vi "Redirection Collection.vi"(8 "error in":errorcluster) -> (0 "error out":errorcluster)   [LabVIEW 2020, in "MainVIs.lvlib"]
uses:
  MainVIs.lvlib
  <vilib>/Utility/miscctls.llb/LVCursorListTypeDef.ctl
  Collection Support/Controls/PED States.ctl
  Collection Support/Controls/FirstCall.ctl
  CollectionSupport.lvlib
panel:
  in  "Delay":u32 max=1000 step=50
  in  "Trial Duration (s)":dbl=10.0 format="%#_13g"
  in  "Max Time":dbl=1.3 min=0.0 max=2.0 format="%#_13g"
  in  "Min Time":dbl=0.8 min=0.0 max=1.0 step=0.1 format="%#_13g"
  in  "Start Second":dbl=2.5 min=1.0 max=2.5 step=0.1 format="%#_13g"
  in  "Interruptions":i32
  in  "Settings":bool
  in  "Restart Button":bool
  in  "Exit Button":bool
  out "Flow Chart":dynamicdata(graph)
  out "Audio Chart":dynamicdata(graph)
  in  "START/STOP":bool
  out "GO/STOP":bool
  out "SPL Chart":cluster{"Y":dbl[], "Y":dbl[]}[](graph)
  out "Countdown":dbl format="%#.0g"
  out "Pressure Chart":dynamicdata(graph)
  in  "Stopped?":bool
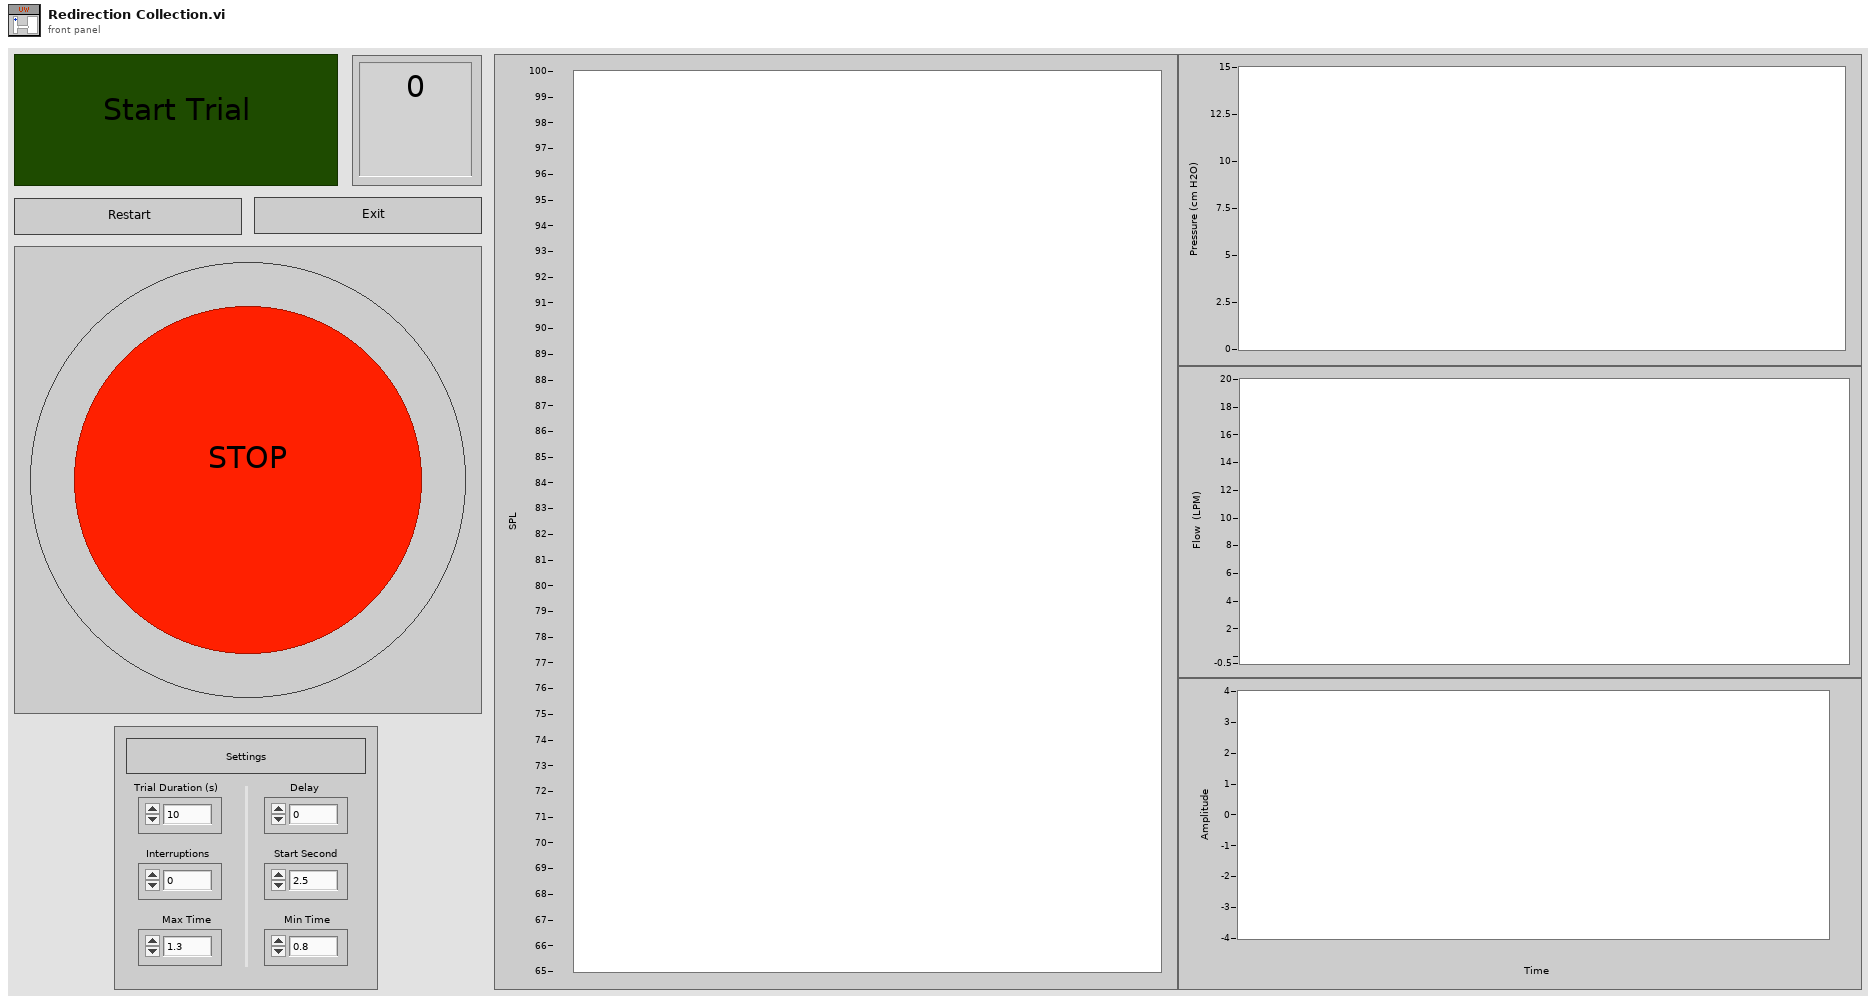
[diagram p1: front panel]
types:
  T1 = enum16{"open", "replace", "create", "open or create", "replace or create", "replace or create with confirmation"}
  T2 = typedef "LVCursorListTypeDef.ctl" = cluster{"Name":string, "Color":u32, "Style":u8, "Point Style":u8, "Name Visible":bool, "Allow Drag":bool, "Cursor Mode":u32, "Plot":i32, "Index":i32, "Position":cluster{"X":dbl, "Y":dbl}, "X Scale":u32, "Y Scale":u32, "Watch Plots":i32[], "Watch All Plots":bool, "Plot Area":i32, "Label Offset":cluster{"X":dbl, "Y":dbl}}[]
  T3 = typedef "CollectionSupport.lvlib/PED States.ctl" = enum16{"Initialize", "Wait", "Record", "Save", "Reset", "Exit"}
  T4 = typedef "CollectionSupport.lvlib/FirstCall.ctl" = enum16{"First", "After"}
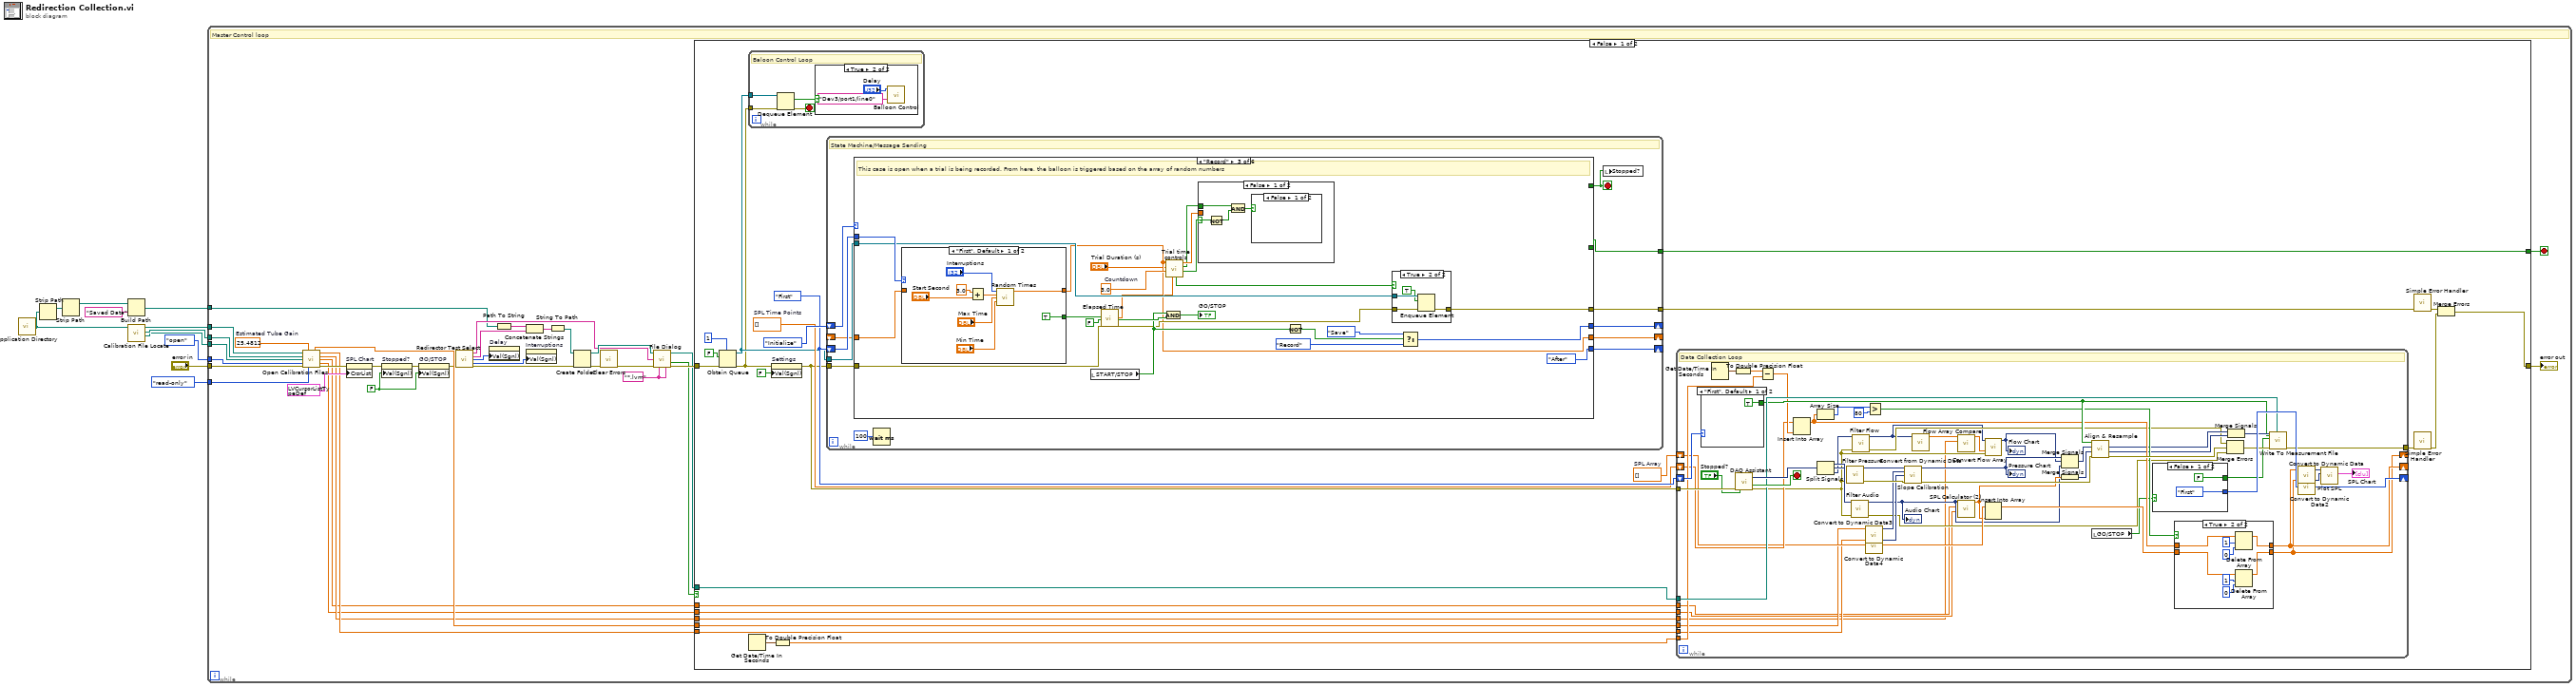
[diagram p0: block diagram]
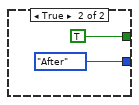
[diagram p4: hidden frame]
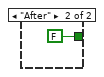
[diagram p5: hidden frame]
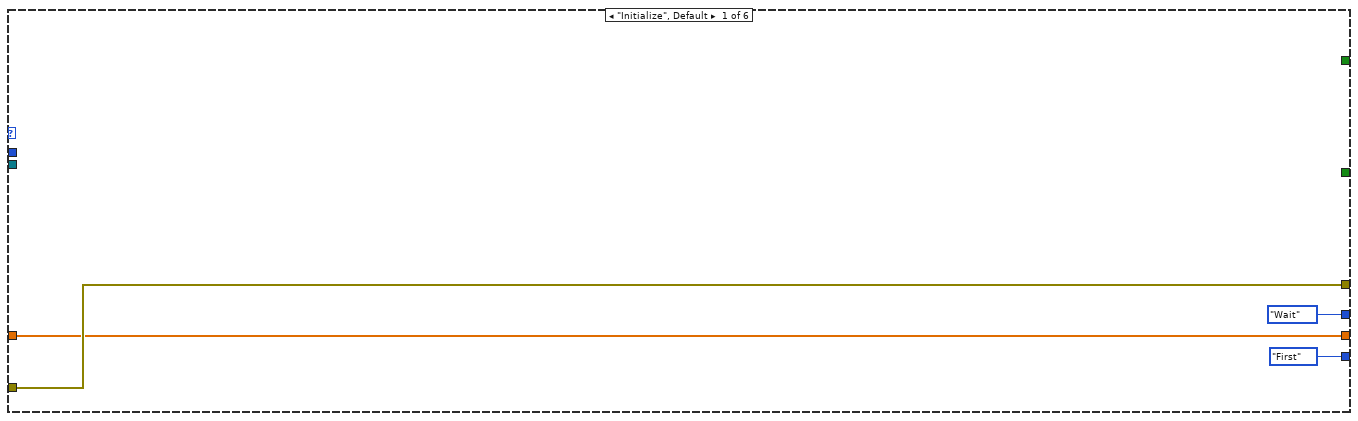
[diagram p6: hidden frame]
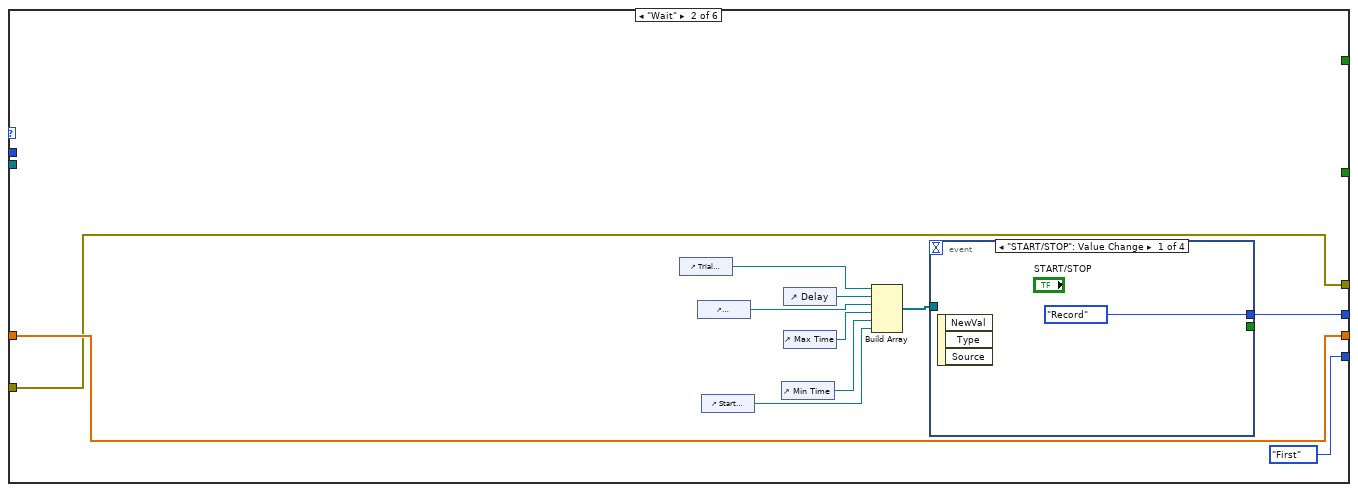
[diagram p7: hidden frame]
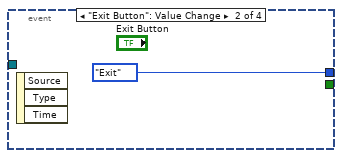
[diagram p8: hidden frame]
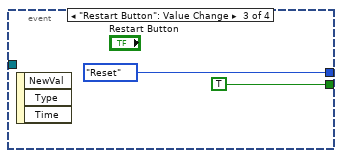
[diagram p9: hidden frame]
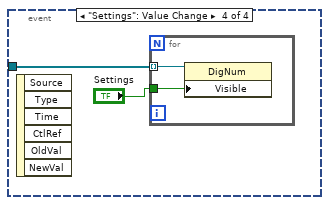
[diagram p10: hidden frame]
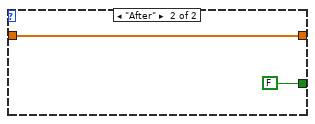
[diagram p12: hidden frame]
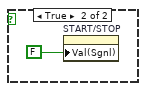
[diagram p13: hidden frame]
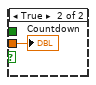
[diagram p14: hidden frame]
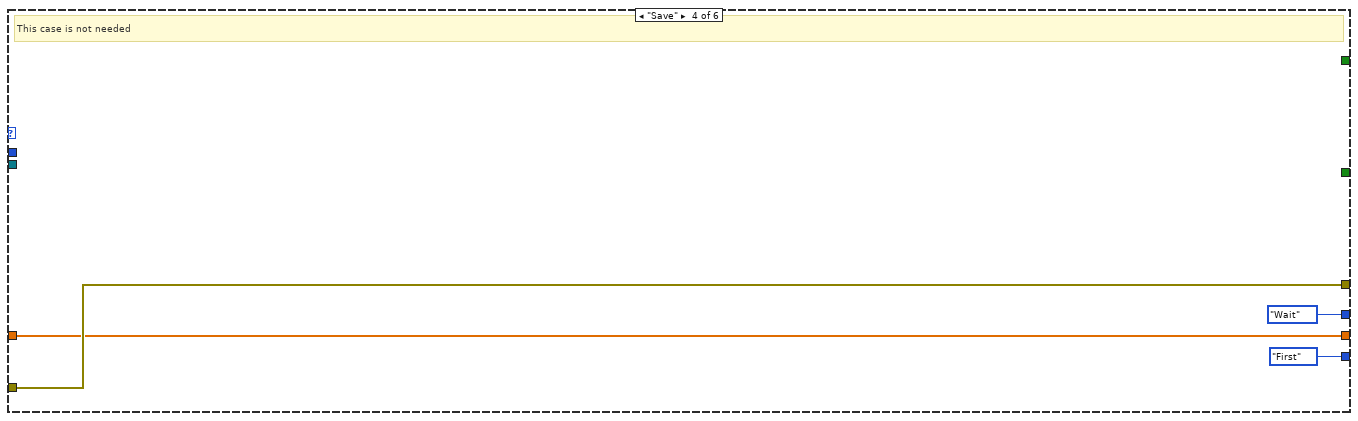
[diagram p15: hidden frame]
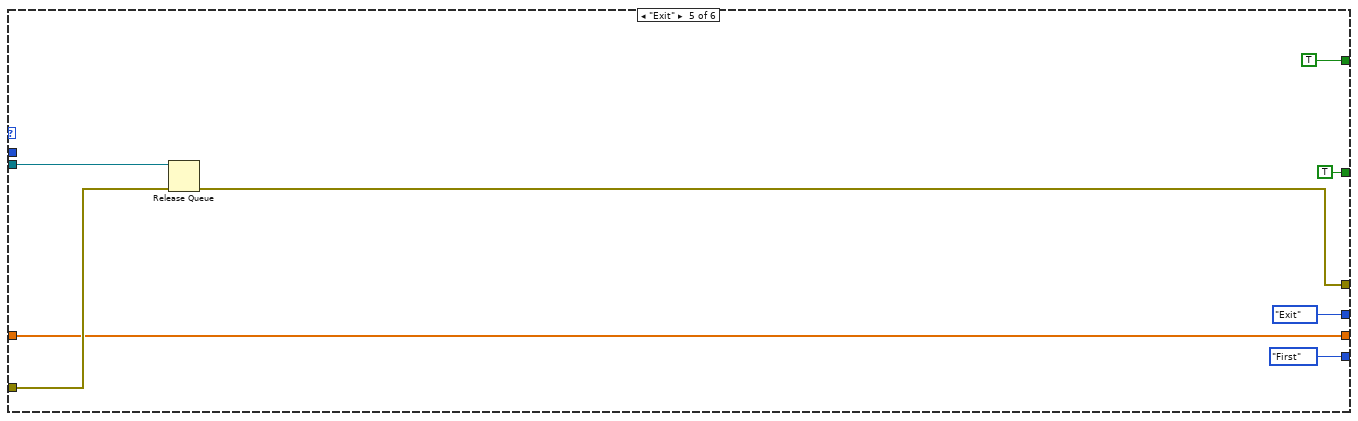
[diagram p16: hidden frame]
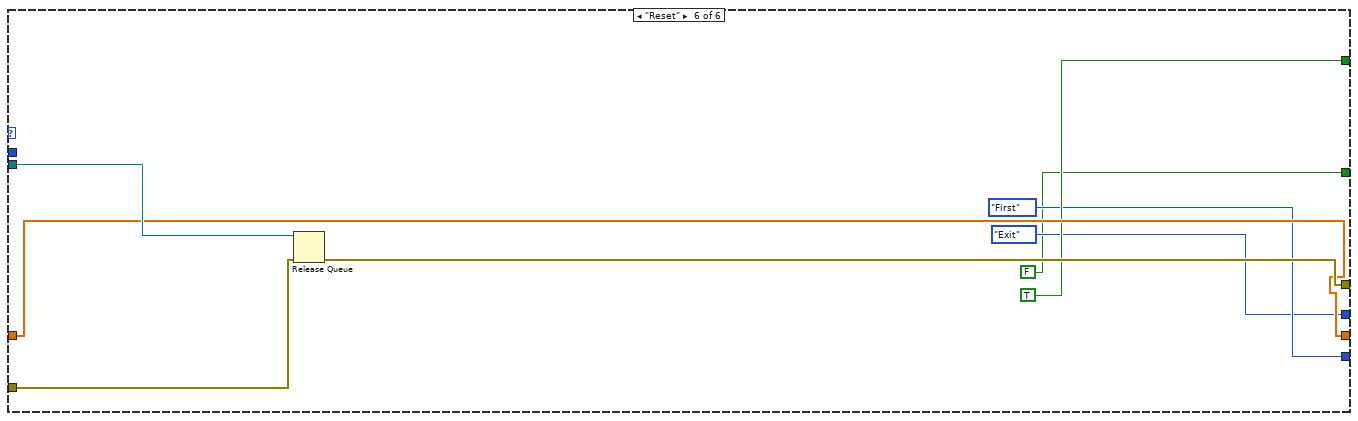
[diagram p17: hidden frame]
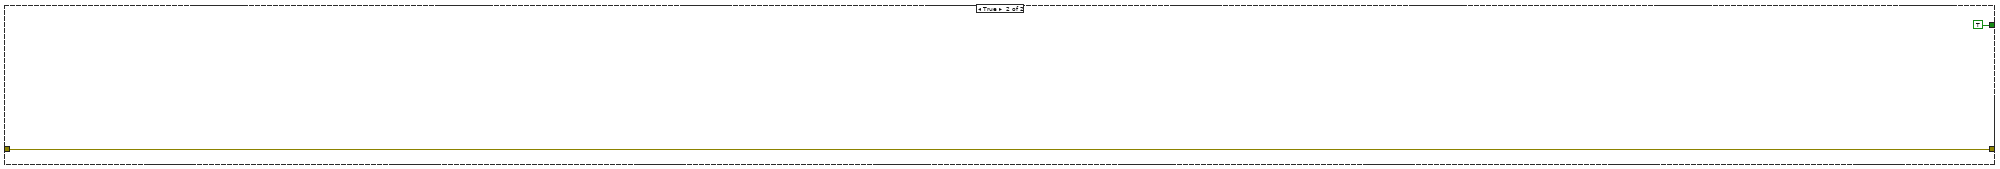
[diagram p18: hidden frame]
diagram:
  n1 = call <vilib>:"Application Directory.vi"() -> ("Application Directory"=w3:path)
  n2 = Strip Path(path=w3) -> (stripped path=w8:path)  [unwired: 1 out]
  n3 = Strip Path(path=w8) -> (stripped path=w2:path)  [unwired: 1 out]
  n4 = Build Path(base path=w2, name or relative path="Saved Data") -> (appended path=w1:path)
  n5 = call "Calibration File Locate.vi"("Base Path"=w3) -> ("SPL Calibration"=w4:path, "Flow Calibration"=w5:path, "Pressure Calibration"=w6:path)  [unwired: 8 in]
  n6 = while {
    tunnel: w5 -> [w41]
    tunnel: T1."open" ("operation (0:open)") -> [w39]
    tunnel: enum16{"read/write", "read-only", "write-only"}."read-only" ("access (0:read/write)") -> [w38]
    tunnel: w6 -> [w42]
    tunnel: w4 -> [w40]
    tunnel: "error in" -> [w36]
    tunnel: w1 -> [w12]
    stop <- w25 stop-if-true
    w37 = 25.4812  # Estimated Tube Gain
    w17 = FALSE ("Value (Signaling)")
    w45 = "*.lvm" ("pattern label")
    # "Master Control loop"
    n7 = call "Open Calibration Files.vi"("Pressure Calibration Path"=w42, "Estimated Tube Gain"=w37, "Flow Array Path"=w41, "SPL Calibration Path"=w40, "operation (0:open)"=w39, "error in (no error)"=w36, "access (0:read/write)"=w38) -> ("Pressure Slope"=w22:dbl, "Pressure Intercept"=w21:dbl, "Flow Array"=w20:dbl[], "Microphone Sensitivity"=w19:dbl, "SPL Gain"=w18:dbl, "error out"=w33:errorcluster)  [unwired: 3 in]
    n8 = property on="SPL Chart" class="XYGraph (strict)"(error in=w33, "CrsrList"=T2 [{"Name"="Upper", "Color"=16860, "Style"=6, "Point Style"=6, "Name Visible"=TRUE, "Allow Drag"=TRUE, "Cursor Mode"=0, "Plot"=0, "Index"=0, "Position"={"X"=4.012670393065205, "Y"=89.47406993320811}, "X Scale"=0, "Y Scale"=0, "Watch Plots"=[], "Watch All Plots"=FALSE, "Plot Area"=0, "Label Offset"={"X"=-0.0013496383482243246, "Y"=198885117671824.3}}, {"Name"="Lower", "Color"=6618880, "Style"=6, "Point Style"=13, "Name Visible"=TRUE, "Allow Drag"=TRUE, "Cursor Mode"=0, "Plot"=0, "Index"=0, "Position"={"X"=1.9573651669874723, "Y"=85.30922361500785}, "X Scale"=0, "Y Scale"=0, "Watch Plots"=[], "Watch All Plots"=FALSE, "Plot Area"=0, "Label Offset"={"X"=0.0011253990502635425, "Y"=1813042855982289.8}}] ("Cursor List")) -> (error out=w32:errorcluster)  [unwired: 1 in, 1 out]
    n9 = property on="Stopped?" class="Bool (strict)"(error in=w32, "Val(Sgnl)"=w17) -> (error out=w16:errorcluster)  [unwired: 1 in, 1 out]
    n10 = property on="GO/STOP" class="Bool (strict)"(error in=w16, "Val(Sgnl)"=w17) -> (error out=w15:errorcluster)  [unwired: 1 in, 1 out]
    n11 = call "Redirector Test Select.vi"("Error In"=w15) -> ("File Name"=w28:string, "Subject Out"=w29:string, "Delay"=w13:u32, "Interruptions"=w14:i32, "Error Out"=w31:errorcluster)  [unwired: 10 in]
    n12 = property on="Delay" class="DigNum (strict)"("Val(Sgnl)"=w13) -> ()  [unwired: 2 in, 2 out]
    n13 = Path To String(path=w12) -> (string=w30:string)
    n14 = Concatenate Strings(w30, w29) -> (w27:string)
    n15 = property on="Interruptions" class="DigNum (strict)"("Val(Sgnl)"=w14) -> ()  [unwired: 2 in, 2 out]
    n16 = String To Path(string=w27) -> (path=w26:path)
    n17 = Create Folder(path (use dialog)=w26, error in=w31) -> (created path=w34:path, error out=w23:errorcluster)  [unwired: 1 in, 1 out]
    n18 = call <vilib>:"Clear Errors.vi"("error in (no error)"=w23) -> ("error out"=w24:errorcluster)  [unwired: 5 in, 1 out]
    n19 = call "File Dialog"("start path"=w34, "default name"=w28, "error in"=w24, "pattern (all files)"=w45, "pattern label"=w45) -> ("selected path"=w46:path, "cancelled"=w43:bool, "error out"=w47:errorcluster)  [unwired: 7 in, 1 out]
    n20 = case shown="False" w43 {
      tunnel: w47 -> [w68 w253]
      tunnel: w46 -> [w67 _]
      tunnel: [w62 w253] -> w44
      tunnel: [w53 TRUE] -> w25
      tunnel: w22 -> [w52 _]
      tunnel: w21 -> [w51 _]
      tunnel: w20 -> [w50 _]
      tunnel: w19 -> [w49 _]
      tunnel: w18 -> [w48 _]
      frame False {
        w58 = dbl[] []  # SPL Array
        w59 = dbl[] []  # SPL Time Points
        w69 = FirstCall."First"
        n21 = Obtain Queue(max queue size (-1, unlimited)=1, element data type=FALSE, error in (no error)=w68) -> (queue out=w57:refnum<queue>, error out=w56:errorcluster)  [unwired: 2 in, 1 out]
        n22 = while {
          tunnel: w57 -> [w76]
          tunnel: w56 -> [w75]
          stop <- w74 stop-if-true
          # "Baloon Control Loop"
          n23 = Dequeue Element(queue=w76, error in (no error)=w75) -> (element=w73:bool, error out=w74:errorcluster)  [unwired: 1 in, 2 out]
          n24 = case shown="True" w73 {
            frame False {
            }
            frame True {
              n25 = call "Balloon Control.vi"("lines"=tag "Dev3/port1/line0", "Delay (ms)"="Delay") -> ()  [unwired: 10 in]
            }
          }
        }
        n26 = Get Date/Time In Seconds() -> (seconds since 1Jan1904=w61:timestamp)
        n27 = property on="Settings" class="Bool (strict)"(error in=w56, "Val(Sgnl)"=FALSE ("Value (Signaling)")) -> (error out=w55:errorcluster)  [unwired: 1 in, 1 out]
        n28 = To Double Precision Float(number=w61) -> (double precision float=w60:dbl)
        n29 = while {
          shift-right: [w163] -> _
          shift-left: PED_States."Initialize" -> [w162]
          tunnel: w57 -> [w159]
          tunnel: w55 -> [w161]
          shift-right: [w158] -> _
          shift-left: w69 -> [w160]
          tunnel: [w156] -> w65
          shift-right: [w153] -> _
          shift-left: _ -> [w154]
          tunnel: [w152] -> w53
          stop <- w157 stop-if-true
          # "State Machine/Message Sending"
          n30 = case shown="\"Record\"" w162 {
            tunnel: [_ _ _ _ TRUE TRUE] -> w157
            tunnel: [PED_States."Wait" ("f") w175 w200 PED_States."Wait" ("element") PED_States."Exit" ("element") PED_States."Exit" ("element")] -> w163
            tunnel: w161 -> [w165 w176 w206 w233 w241 w250]
            tunnel: w160 -> [_ _ w202 _ _ _]
            tunnel: w159 -> [_ _ w198 _ w240 w249]
            tunnel: [FirstCall."First" FirstCall."First" FirstCall."After" FirstCall."First" FirstCall."First" FirstCall."First"] -> w158
            tunnel: [w164 w177 w193 w232 w237 w248] -> w153
            tunnel: [w165 w176 w197 w233 w238 w251] -> w156
            tunnel: w154 -> [w164 w177 w196 w232 w237 w248]
            tunnel: [_ _ _ _ TRUE FALSE] -> w152
            frame "Initialize", Default {
            }
            frame "Wait" {
              n31 = control-ref of="Trial Duration (s)"() -> (w173:refnum<vi>)
              n32 = control-ref of="Interruptions"() -> (w171:refnum<vi>)
              n33 = control-ref of="Start Second"() -> (w168:refnum<vi>)
              n34 = control-ref of="Min Time"() -> (w169:refnum<vi>)
              n35 = control-ref of="Delay"() -> (w172:refnum<vi>)
              n36 = control-ref of="Max Time"() -> (w170:refnum<vi>)
              n37 = Build Array(w173, w172, w171, w170, w169, w168) -> (w174:refnum<vi>[])
              n38 = event shown="[0] \"START/STOP\": Value Change" {
                selector: _ -> [_ _ _ _]
                dyn-events: _ -> [_ _ _ _]
                timeout: _ -> [_ _ _ _]
                tunnel: [PED_States."Record" ("element") PED_States."Exit" ("element") PED_States."Reset" ("element") _] -> w175
                tunnel: [_ _ TRUE _] -> _
                tunnel: w174 -> [_ _ _ w184]
                event "START/STOP": Value Change {
                  n39 = event-data() -> ()  [unwired: 1 in, 3 out]
                }
                event "Exit Button": Value Change {
                  n40 = event-data() -> ()  [unwired: 1 in, 3 out]
                }
                event "Restart Button": Value Change {
                  n41 = event-data() -> ()  [unwired: 1 in, 3 out]
                }
                event "Settings": Value Change {
                  n42 = event-data() -> ()  [unwired: 1 in, 6 out]
                  n43 = for {
                    tunnel: w184 -> [w186] mode=indexing
                    tunnel: "Settings" -> [w185]
                    n44 = property class="DigNum"(reference=w186, "Visible"=w185) -> ()  [unwired: 1 in, 2 out]
                  }
                }
              }
            }
            frame "Record" {
              w194 = 3.0  # Countdown
              # "This case is open when a trial is being recorded. From here, the balloon is triggered based on the array of random numbers"
              n45 = case shown="\"First\", Default" w202 {
                tunnel: [TRUE FALSE] -> w203
                tunnel: [w222 w224] -> w193
                tunnel: w196 -> [_ w224]
                frame "First", Default {
                  n46 = Add(x=3.0, y="Start Second") -> (x+y=w218:dbl)
                  n47 = call "Random Times.vi"("Number of Interruptions"="Interruptions", "Start Second"=w218, "Longest Gap"="Max Time", "Shortest Gap"="Min Time") -> ("Interruption TImes"=w222:dbl[])  [unwired: 10 in, 1 out]
                }
                frame "After" {
                }
              }
              n48 = local read "START/STOP"() -> (w207:bool)
              n49 = call "Elapsed Time"("Reset"=w203, "Auto Reset"=FALSE, "error in (no error)"=w206) -> ("Elapsed Time (s)"=w189:dbl, "Time has Elapsed"=w208:bool, "error out"=w199:errorcluster)  [unwired: 9 in, 5 out]
              n50 = And(x=w207, y=w208) -> (x .and. y?=→"GO/STOP":bool)
              n51 = call "Trial time controls.vi"("Elapsed Time (s)"=w189, "Countdown"=w194, "Trial Duration (s)"="Trial Duration (s)", "Interruption Times"=w193) -> ("End of Countdown?"=w190:bool, "Trial Complete?"=w191:bool, "Countdown"=w192:dbl, "Trigger Balloon?"=w188:bool)  [unwired: 4 in]
              n52 = case shown="False" w190 {
                selector: w190 -> [w228 _]
                tunnel: w192 -> [_ w231]
                tunnel: w191 -> [w226 _]
                frame False {
                  n53 = Not(x=w228) -> (.not. x?=w227:bool)
                  n54 = And(x=w226, y=w227) -> (x .and. y?=w229:bool)
                  n55 = case shown="False" w229 {
                    frame False {
                    }
                    frame True {
                      n56 = property on="START/STOP" class="Bool (strict)"("Val(Sgnl)"=FALSE ("Value (Signaling)")) -> ()  [unwired: 2 in, 2 out]
                    }
                  }
                }
                frame True {
                  "Countdown" <- w231
                }
              }
              n57 = Not(x=w207) -> (.not. x?=w205:bool)
              n58 = case shown="True" w188 {
                tunnel: [w211 w215] -> w197
                tunnel: w199 -> [w211 w214]
                tunnel: w198 -> [_ w213]
                frame False {
                }
                frame True {
                  n59 = Enqueue Element(queue=w213, element=TRUE, error in (no error)=w214) -> (error out=w215:errorcluster)  [unwired: 1 in, 2 out]
                }
              }
              n60 = Select(t=PED_States."Save" ("f"), s=w205, f=PED_States."Record") -> (s? t:f=w200:T3)
            }
            frame "Save" {
              # "This case is not needed"
            }
            frame "Exit" {
              n61 = Release Queue(queue=w240, error in (no error)=w241) -> (error out=w238:errorcluster)  [unwired: 1 in, 2 out]
            }
            frame "Reset" {
              n62 = Release Queue(queue=w249, error in (no error)=w250) -> (error out=w251:errorcluster)  [unwired: 1 in, 2 out]
            }
          }
          n63 = Wait (ms)(milliseconds to wait=u32 100) -> ()  [unwired: 1 out]
          n64 = local write "Stopped?"(w157) -> ()
        }
        n65 = while {
          tunnel: w55 -> [w129]
          shift-right: [w125] -> _
          shift-left: w69 -> [w126]
          tunnel: w67 -> [w124]
          tunnel: [w120] -> w66
          tunnel: w60 -> [w115]
          shift-right: [w103] -> _
          shift-left: w59 -> [w113]
          shift-right: [w102] -> _
          shift-left: w58 -> [w104]
          tunnel: w52 -> [w98]
          tunnel: w51 -> [w97]
          tunnel: w50 -> [w79]
          tunnel: w49 -> [w85]
          tunnel: w48 -> [w84]
          stop <- w130 stop-if-true
          # "Data Collection Loop"
          n66 = case shown="\"First\", Default" w126 {
            tunnel: [TRUE FALSE] -> w118
            frame "First", Default {
            }
            frame "After" {
            }
          }
          n67 = Get Date/Time In Seconds() -> (seconds since 1Jan1904=w117:timestamp)
          n68 = To Double Precision Float(number=w117) -> (double precision float=w116:dbl)
          n69 = call "DAQ Assistant"("error in"=w129, "stop (F)"="Stopped?") -> ("data"=w133:dynamicdata, "stopped"=w130:bool, "error out"=w83:errorcluster)  [unwired: 14 in, 1 out]
          n70 = Subtract(x=w116, y=w115) -> (x-y=w114:dbl)
          n71 = Insert Into Array(array=w113, new element=w114) -> (w105:dbl[])  [unwired: 1 in]
          n72 = Array Size(array=w105) -> (size(s)=w111:i32)
          n73 = Split Signals(w133) -> (w134:dynamicdata, w119:dynamicdata, w96:dynamicdata)  [unwired: 3 in]
          n74 = call "Filter Pressure"("error in (no error)"=w83, "Signal"=w119) -> ("error out"=w132:errorcluster, "Filtered Signal"=w135:dynamicdata)  [unwired: 8 in]
          n75 = call "Filter Audio"("error in (no error)"=w83, "Signal"=w134) -> ("error out"=w87:errorcluster, "Filtered Signal"=w86:dynamicdata)  [unwired: 8 in]
          "Audio Chart" <- w86
          n76 = call "Filter Flow"("error in (no error)"=w83, "Signal"=w96) -> ("error out"=w82:errorcluster, "Filtered Signal"=w81:dynamicdata)  [unwired: 8 in]
          n77 = call "Convert to Dynamic Data3"("Double"=w98) -> ("Dynamic Data Type"=w100:dynamicdata)  [unwired: 3 in]
          n78 = call "Convert to Dynamic Data4"("Double"=w97) -> ("Dynamic Data Type"=w99:dynamicdata)  [unwired: 3 in]
          n79 = Greater?(x=w111, y=80) -> (0:w108:bool)
          n80 = call "Slope Calibration.vi"("Voltage"=w135, "Slope"=w100, "Intercept"=w99, "error in (no error)"=w132) -> ("Result"=w94:dynamicdata, "error out"=w131:errorcluster)  [unwired: 10 in]
          "Pressure Chart" <- w94
          n81 = call "Convert from Dynamic Data"("Dynamic Data Type"=w81) -> ("Array"=w80:dbl[])  [unwired: 3 in]
          n82 = call "Flow Array Compare.vi"("Flow Array in"=w79, "Array in"=w80) -> ("Array out"=w95:dbl[])  [unwired: 9 in]
          n83 = call "SPL Calculator (2).vi"("Gain"=w84, "Microphone Sensitvity (dBV/Pa)"=w85, "Filtered Signal"=w86) -> ("SPL"=w91:dbl)  [unwired: 7 in, 1 out]
          n84 = call "Convert Flow Array.vi"("Voltage"=w81, "Array - Numeric"=w95, "error in (no error)"=w83) -> ("Result"=w93:dynamicdata)  [unwired: 11 in, 1 out]
          "Flow Chart" <- w93
          n85 = Insert Into Array(array=w104, new element=w91) -> (w107:dbl[])  [unwired: 1 in]
          n86 = Merge Signals(w94, w93, w86) -> (w92:dynamicdata)
          n87 = Merge Signals(w91) -> (w90:dynamicdata)
          n88 = call "Align & Resample"("error in (no error)"=w131, "Signals 2"=w90, "Signals"=w92, "Reset"=w118) -> ("error out"=w127:errorcluster, "Resampled Signals 2"=w88:dynamicdata, "Resampled Signals"=w89:dynamicdata)  [unwired: 5 in]
          n89 = local read "GO/STOP"() -> (w101:bool)
          n90 = case shown="False" w101 {
            tunnel: [FirstCall."First" FirstCall."After"] -> w125
            tunnel: [FALSE TRUE] -> w121
            frame False {
            }
            frame True {
            }
          }
          n91 = case shown="True" w108 {
            tunnel: w107 -> [w137 w145]
            tunnel: [w137 w144] -> w102
            tunnel: w105 -> [w136 w139]
            tunnel: [w136 w138] -> w103
            frame False {
            }
            frame True {
              n92 = Delete From Array(array=w139, length=1, index=0) -> (array with subset deleted=w138:dbl[])  [unwired: 1 out]
              n93 = Delete From Array(array=w145, length=1, index=0) -> (array with subset deleted=w144:dbl[])  [unwired: 1 out]
            }
          }
          n94 = Merge Errors(w82, w127, w87) -> (w122:errorcluster)
          n95 = Merge Signals(w89, w88) -> (w123:dynamicdata)
          n96 = call "Write To Measurement File"("Signals"=w123, "Reset"=w118, "Enable"=w121, "error in (no error)"=w122, "Filename"=w124) -> ("error out"=w120:errorcluster)  [unwired: 12 in, 2 out]
          n97 = call "Convert to Dynamic Data"("Array"=w103) -> ("Dynamic Data Type"=w109:dynamicdata)  [unwired: 3 in]
          n98 = call "Convert to Dynamic Data2"("Array"=w102) -> ("Dynamic Data Type"=w110:dynamicdata)  [unwired: 3 in]
          n99 = call "Plot SPL"("Y Input"=w110, "X Input"=w109) -> ("XY Graph"=→"SPL Chart":cluster{"Y":dbl[], "Y":dbl[]}[])  [unwired: 8 in, 1 out]
        }
        n100 = call <vilib>:"Simple Error Handler.vi"("error in (no error)"=w65) -> ("error out"=w64:errorcluster)  [unwired: 4 in, 4 out]
        n101 = call <vilib>:"Simple Error Handler.vi"("error in (no error)"=w66) -> ("error out"=w63:errorcluster)  [unwired: 4 in, 4 out]
        n102 = Merge Errors(w64, w63) -> (w62:errorcluster)
      }
      frame True {
      }
    }
    "error out" <- w44
  }
